vi "ActionVIOnCompile.vi"(8 "error in":errorcluster, 11 "Device Item Ref in":u64 format="%.0x") -> (0 "error out":errorcluster)   [LabVIEW 2026, in "Template Configuration.lvlib"]
uses:
  Template Configuration.lvlib
  <vilib>/NI VeriStand/Custom Device API/Set Item Property (Variant).vi
  NationalInstruments.VeriStand.SystemDefinitionAPI
  <userlib>/Custom Device Interfaces_v1.lvlibp/CustomDeviceDeploymentHooks/Custom Device Deployment Hooks.lvclass
  <vilib>/NI VeriStand/Custom Device API/Custom Device API.lvlib
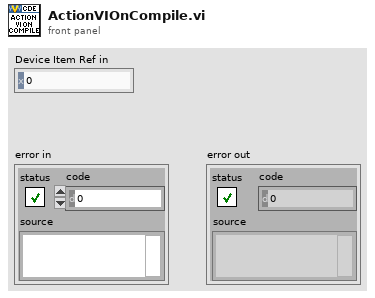
[diagram p1: front panel]
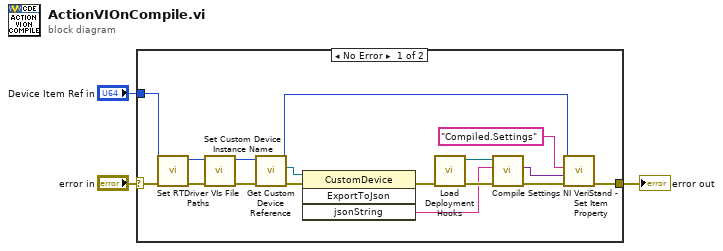
[diagram p0: block diagram]
diagram:
  n1 = case shown="No Error" "error in" {
    selector: "error in" -> [w20 w21]
    tunnel: [w10 w21] -> w2
    tunnel: "Device Item Ref in" -> [w19 _]
    frame No Error {
      n2 = call "Set RTDriver VIs File Paths.vi"("error in"=w20, "Item Ref in"=w19) -> ("error out"=w16:errorcluster, "Item Ref out"=w12:u64)  [unwired: 8 in]
      n3 = call "Set Custom Device Instance Name.vi"("error in"=w16, "Item Ref in"=w12) -> ("error out"=w4:errorcluster, "Item Ref out"=w8:u64)  [unwired: 8 in]
      n4 = call "Get Custom Device Reference.vi"("error in"=w4, "Item Ref in"=w8) -> ("error out"=w5:errorcluster, "Custom Device"=w6:refnum<k24>, "Item Ref out"=w7:u64)  [unwired: 7 in]
      n5 = invoke class="CustomDevice" method="ExportToJson"(reference=w6, error in=w5) -> (error out=w11:errorcluster, "jsonString"=w9:string)  [unwired: 2 in, 2 out]
      n6 = call "Load Deployment Hooks.vi"("error in"=w11) -> ("error out"=w18:errorcluster, "Custom Device Deployment Hooks out"=w14:refnum<class "Custom Device Deployment Hooks.lvclass">)  [unwired: 9 in]
      n7 = call-dynamic "Compile Settings.vi"("error in"=w18, "Settings(JSON)"=w9, "Custom Device Deployment Hooks in"=w14) -> ("error out"=w17:errorcluster, "Compiled Settings"=w13:variant)  [unwired: 6 in, 1 out]
      n8 = call-poly <vilib>:"NI VeriStand - Set Item Property.vi"("error in (no error)"=w17, "Value"=w13, "Property Name"="Compiled.Settings" ("Compiled.Settings"), "Item Ref in"=w7) -> ("error out"=w10:errorcluster)  [unwired: 5 in, 2 out]
    }
    frame Error {
    }
  }
  "error out" <- w2
